vi "delete_zeros.vi"(10 "array_in":u32[](array[numeric])) -> (2 "array_out":u32[](array[numeric]))   [LabVIEW 2018]
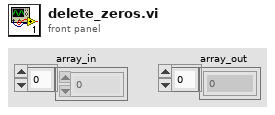
[diagram p1: front panel]
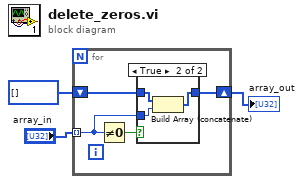
[diagram p0: block diagram]
diagram:
  n1 = for {
    tunnel: "array_in" -> [w4] mode=indexing
    shift-right: [w5] -> w3
    shift-left: u32[] [] ("array_in") -> [w6]
    n2 = Not Equal To 0?(x=w4) -> (x != 0?=w7:bool)
    n3 = case shown="True" w7 {
      tunnel: w6 -> [w8 w11]
      tunnel: [w8 w10] -> w5
      tunnel: w4 -> [_ w9]
      frame False {
      }
      frame True {
        n4 = Build Array (concatenate)(w11, w9) -> (w10:u32[])
      }
    }
  }
  "array_out" <- w3
